vi "Battery First Match Test.vi"() -> ()   [LabVIEW 2014]
uses:
  Controls/PC Data.ctl
  Controls/MicroZed Config Op Mode.ctl
  Controls/ES System Data.ctl
  Controls/StringSelector.ctl
  Controls/ES String Array.ctl
  Controls/ES String Data.ctl
panel:
  out "Precharge Current Out":sgl
  out "ES ON Array Out":bool[](array[boolean])
  out "Matching Complete":bool=TRUE
  in  "ES String Data":T1
  in  "ES System Data":T3={"Voltage"=0.0, "Current"=0.0, "SOC Avg"=0.0, "Faults"=0, "Alarms"=0, "# Strings"=0, "Max Temp"=0, "Min Temp"=0, "Max Cell Voltage"=0.0, "Min Cell Voltage"=0.0, "Energy Capacity"=0.0, "Energy Remaining"=0.0, "SOC Min"=0.0, "SOC Max"=0.0, "ES Fault"=FALSE, "String Select"=enum."3 Strings", "ES Com Fault"=FALSE, "SOH Avg"=0.0}
  in  "PC Data":T5 {"Alarms 2" format="%016b"; "Faults 2" format="%016b"; "Alarms 1" format="%016b"; "Faults 1" format="%016b"; "Contactor FB" format="%.0b"; "DC Voltage SP" format="%2.1f"; "Clear Faults SP" format="%.0b"; "Neutral Current" format="%2.1f"; "AC Current - L2" format="%2.1f"; "AC Voltage - L2" format="%2.1f"; "Temperature" format="%2.1f"; "DC Voltage" format="%2.1f"; "AC Current SP" format="%2.1f"; "AC Voltage SP" format="%2.1f"; "Frequency SP" format="%2.1f"; "AC Frequency" format="%2.1f"; "AC Current - L1" format="%2.1f"; "AC Voltage- L1" format="%2.1f"}
  in  "Init":bool
  in  "ES ON Array In":bool[](array[boolean])=[FALSE, FALSE, FALSE, FALSE, FALSE, FALSE, FALSE, FALSE, FALSE, FALSE]
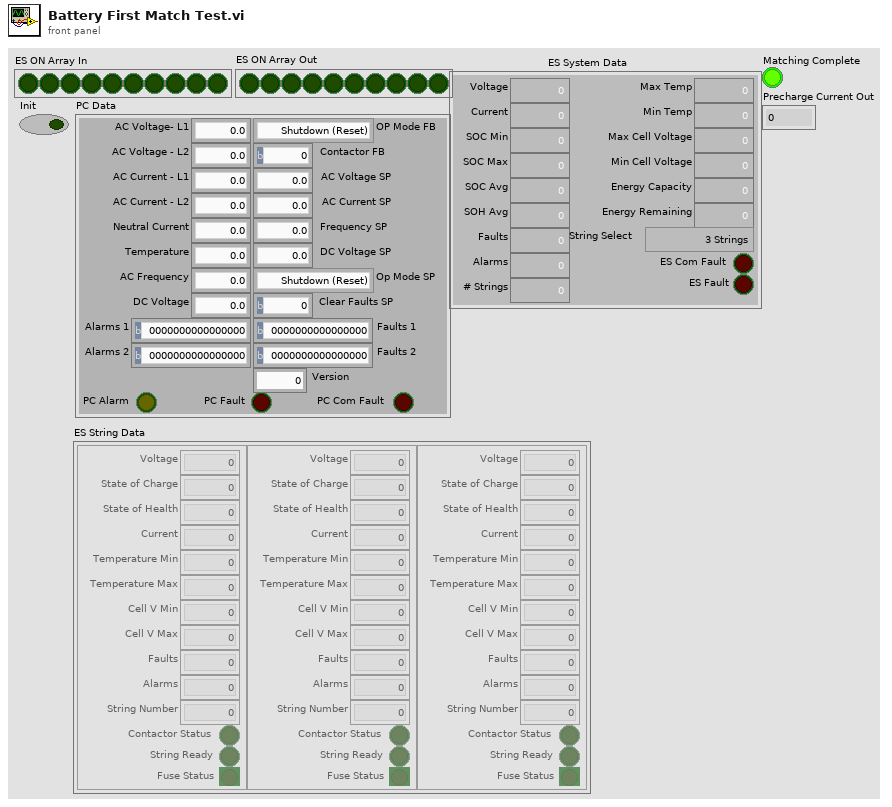
[diagram p1: front panel]
types:
  T1 = typedef "ES String Array.ctl" = T2[]
  T2 = typedef "ES String Data.ctl" = cluster{"Voltage":sgl, "State of Charge":sgl, "Current":sgl, "Temperature Min":i16, "Temperature Max":i16, "Faults":u16, "Alarms":u16, "String Number":u16, "Contactor Status":bool, "String Ready":bool, "Fuse Status":bool, "Cell V Max":dbl, "Cell V Min":dbl, "State of Health":sgl}
  T3 = typedef "ES System Data.ctl" = cluster{"Voltage":sgl, "Current":sgl, "SOC Avg":sgl, "Faults":u16, "Alarms":u16, "# Strings":u16, "Max Temp":i16, "Min Temp":i16, "Max Cell Voltage":sgl, "Min Cell Voltage":sgl, "Energy Capacity":sgl, "Energy Remaining":sgl, "SOC Min":sgl, "SOC Max":sgl, "ES Fault":bool, "String Select":T4, "ES Com Fault":bool, "SOH Avg":sgl}
  T4 = typedef "StringSelector.ctl" = enum16{"1 String (1)", "1 String (2)", "1 String (3)", "2 Strings (1 2)", "2 Strings (2 3)", "2 Strings (1 3)", "3 Strings"}
  T5 = typedef "PC Data.ctl" = cluster{"AC Voltage- L1":dbl, "AC Voltage - L2":dbl, "AC Current - L1":dbl, "AC Current - L2":dbl, "Neutral Current":dbl, "Temperature":dbl, "AC Frequency":dbl, "DC Voltage":dbl, "AC Voltage SP":dbl, "AC Current SP":dbl, "Frequency SP":dbl, "Op Mode SP":T6, "Clear Faults SP":u16, "PC Com Fault":bool, "PC Fault":bool, "DC Voltage SP":dbl, "OP Mode FB":T6, "Contactor FB":u16, "Faults 1":u16, "Alarms 1":u16, "Faults 2":u16, "Alarms 2":u16, "PC Alarm":bool, "Version":u16}
  T6 = typedef "MicroZed Config Op Mode.ctl" = enum16{"Shutdown (Reset)", "Startup", "Idle", "Voltage Mode", "Current Mode", "Fault", "OL Voltage (Debug)", "No Data"}
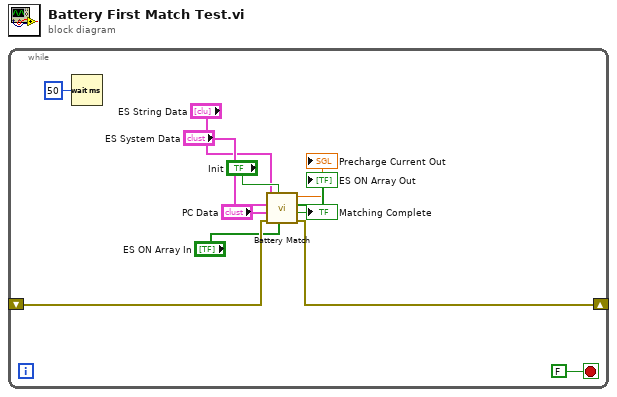
[diagram p0: block diagram]
diagram:
  n1 = while {
    shift-right: [w9] -> _
    shift-left: _ -> [w10]
    stop <- FALSE stop-if-true
    n2 = Wait (ms)(milliseconds to wait=u32 50) -> ()  [unwired: 1 out]
    n3 = call "Battery Match.vi"("ES ON Array In"="ES ON Array In", "Init"="Init", "Error In"=w10, "PC Data"="PC Data", "ES System Data"="ES System Data", "ES String Data"="ES String Data") -> ("Error Out"=w9:errorcluster, "Matching Complete"=→"Matching Complete":bool, "ES ON Array Out"=→"ES ON Array Out":bool[], "Precharge Current Out"=→"Precharge Current Out":sgl)  [unwired: 2 in]
  }
